vi "Saturatio current for solar cell (SubVI).vi"(10 "I_rs":dbl, 11 "T":dbl) -> (3 "I_0":dbl)   [LabVIEW 2024]
panel:
  # "I_0 = I_rs.(T/T_n)^3.exp[(q.E_go.(1/T_n- 1/T))/n.K]"
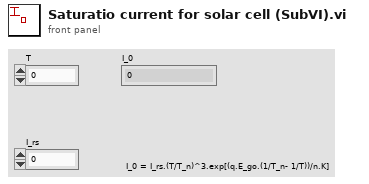
[diagram p1: front panel]
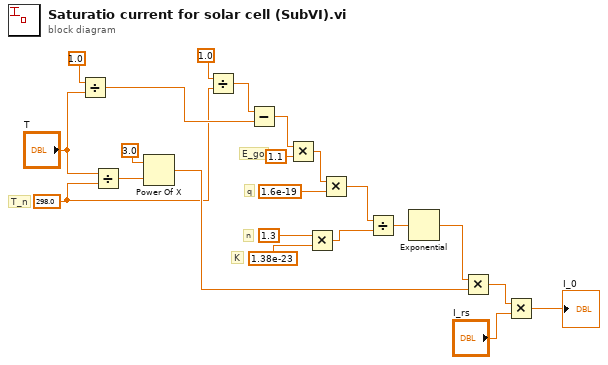
[diagram p0: block diagram]
diagram:
  w5 = 298.0 ("y")
  # "K"
  # "n"
  # "q"
  # "E_go"
  # "T_n"
  n1 = Divide(x=1.0, y="T") -> (x/y=w8:dbl)
  n2 = Divide(x="T", y=w5) -> (x/y=w1:dbl)
  n3 = Power Of X(1:w1, 2:3.0 ("y")) -> (0:w19:dbl)
  n4 = Divide(x=1.0, y=w5) -> (x/y=w7:dbl)
  n5 = Subtract(x=w7, y=w8) -> (x-y=w11:dbl)
  n6 = Multiply(x=w11, y=1.1) -> (x*y=w10:dbl)
  n7 = Multiply(x=1.3 ("y"), y=1.38e-23) -> (x*y=w15:dbl)
  n8 = Multiply(x=w10, y=1.6e-19) -> (x*y=w16:dbl)
  n9 = Divide(x=w16, y=w15) -> (x/y=w17:dbl)
  n10 = Exponential(1:w17) -> (0:w18:dbl)
  n11 = Multiply(x=w18, y=w19) -> (x*y=w20:dbl)
  n12 = Multiply(x=w20, y="I_rs") -> (x*y=→"I_0":dbl)
